vi "Dispatch PVMonitors.vi"(8 "Error In":errorcluster, 11 "CS++ControllerActor in":refnum<class "CS++ControllerActor.lvclass">) -> (0 "Error Out":errorcluster, 3 "CS++ControllerActor out":refnum<class "CS++ControllerActor.lvclass">)   [LabVIEW 2014, in "CS++ControllerActor.lvlib" / "CS++ControllerActor.lvclass"]
doc: "Dispatch nested PVMonitor actors according to PV protocoll prefix."
uses:
  CS++ControllerActor.lvclass
  CS++PVMonitor/CS++PVMonitor.lvclass
  CS++GUIActor Messages/Update-PV Msg/Update-PV Msg.lvclass
  CS++BaseActor/CS++BaseActor.lvclass/CS++BaseActor.ctl
  CS++PVMonitor Messages/CS++PVUpdate Msg/CS++PVUpdate Msg.lvclass/CS++PVUpdate Msg.ctl
  Classes/CS++ProcessVariables/ProcessVariable/PV.lvclass/PV.ctl
  Libraries/Base/FGV Action.ctl
  <vilib>/ActorFramework/Actor/Actor.lvclass/Actor.ctl
  <vilib>/ActorFramework/Message Enqueuer/Message Enqueuer.lvclass/Message Enqueuer.ctl
  CS++ControllerActor.lvclass/CS++ControllerActor.ctl
  CS++PVMonitor Messages/Register PVs Msg/Register PVs Msg.lvclass/Register PVs Msg.ctl
  <vilib>/ActorFramework/Message Enqueuer/Init from Existing Queue.vi
  <vilib>/ActorFramework/Message Enqueuer/Enqueue.vi
  <vilib>/ActorFramework/Message Priority Queue/Priority Enqueue.vi
  CS++PVMonitor Messages/CS++PVUpdate Msg/CS++PVUpdate Msg.lvclass
  Classes/CS++ProcessVariables/PVConnection/PVConnection.lvclass
  Classes/CS++ProcessVariables/ProcessVariable/PV.lvclass
  <vilib>/ActorFramework/Message Enqueuer/Message Enqueuer.lvclass
  CS++PVMonitor Messages/Register PVs Msg/Register PVs Msg.lvclass
  CS++BaseActor/CS++BaseActor.lvclass
  <vilib>/ActorFramework/Actor/Actor.lvclass
  Libraries/Base/CS++Base.lvlib
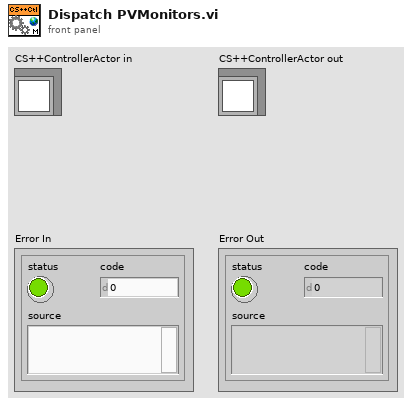
[diagram p1: front panel]
types:
  T1 = cluster{"Msgs":refnum<class "Update-PV Msg.lvclass">[]}[]
  T2 = typedef "CS++Base.lvlib/FGV Action.ctl" = enum16{"add", "replace", "read", "remove", "reset", "get attributes"}
  T3 = cluster{"Name":string, "Polling-String":string, "CS++PVUpdate Msg":refnum<class "CS++PVUpdate Msg.lvclass">, "PVConnection":refnum<class "PVConnection.lvclass">}[]
  T4 = cluster{"Msgs":refnum<class "CS++PVUpdate Msg.lvclass">[]}
  T5 = cluster{"Msgs":refnum<class "CS++PVUpdate Msg.lvclass">[]}[]
  T6 = cluster{refnum<class "CS++PVUpdate Msg.lvclass">[]}
  T7 = cluster{"Accessors:Device Actor's Enqueuer":refnum<class "Message Enqueuer.lvclass">, "Msgs":refnum<class "CS++PVUpdate Msg.lvclass">[]}
  T8 = cluster{"Self Enqueuer":refnum<class "Message Enqueuer.lvclass">, "Msgs":refnum<class "CS++PVUpdate Msg.lvclass">[]}
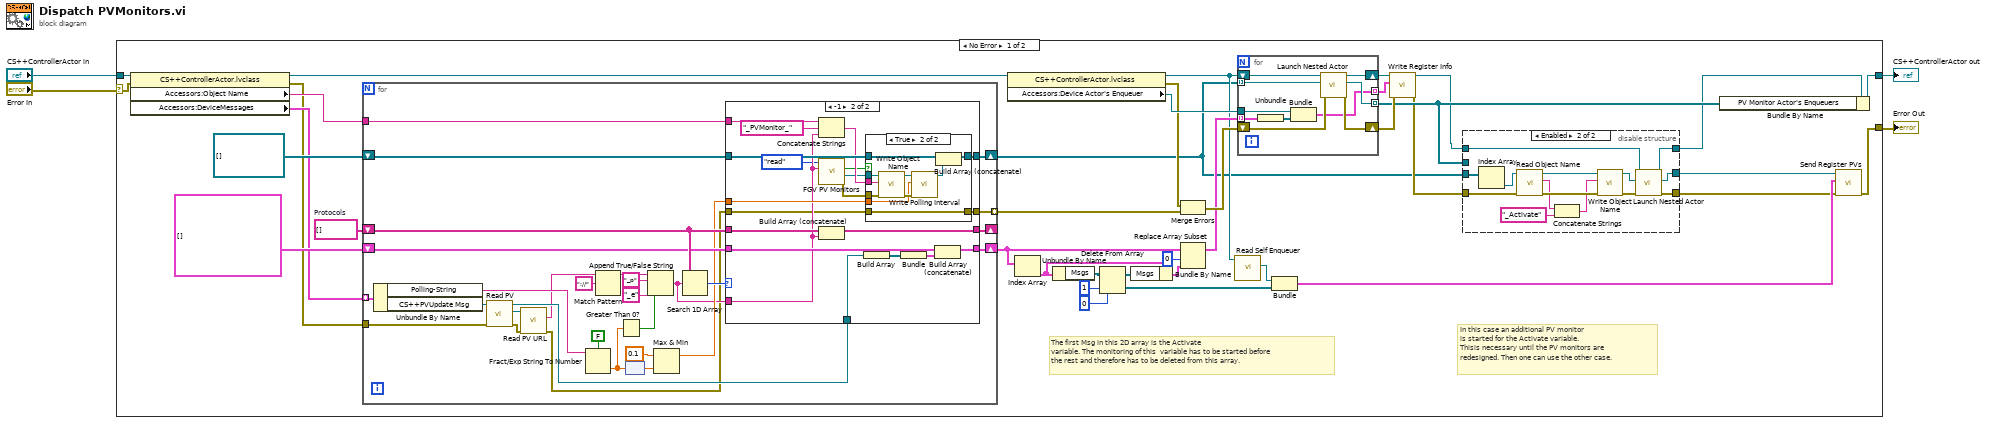
[diagram p0: block diagram]
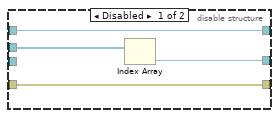
[diagram p2: hidden frame]
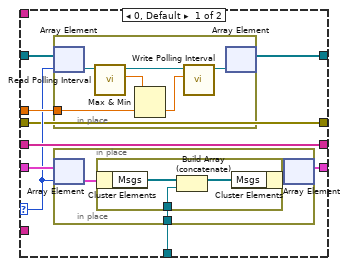
[diagram p3: hidden frame]
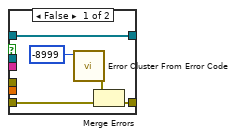
[diagram p4: hidden frame]
diagram:
  n1 = case shown="No Error" "Error In" {
    selector: "Error In" -> [w40 w157]
    tunnel: [w26 w157] -> w3
    tunnel: [w41 w156] -> w1
    tunnel: "CS++ControllerActor in" -> [w42 w156]
    frame No Error {
      w38 = string[] []  # Protocols
      # "In this case an additional PV monitor\nis started for the Activate variable.\nThisis necessary until the PV monitors are\nredesigned. Then one can use the other case."
      # "The first Msg in this 2D array is the Activate\nvariable. The monitoring of this  variable has to be started before\nthe rest and therefore has to be deleted from this array."
      n2 = property class="CS++ControllerActor.lvclass"(reference=w42, error in=w40) -> (reference out=w31:refnum<class "CS++ControllerActor.lvclass">, error out=w29:errorcluster, "Accessors:Object Name"=w34:string, "Accessors:DeviceMessages"=w30:T3)
      n3 = for {
        shift-right: [w99] -> w5
        shift-left: refnum<class "CS++PVMonitor.lvclass">[] [] -> [w96]
        shift-right: [w98] -> _
        shift-left: w38 -> [w97]
        tunnel: w34 -> [w95]
        shift-right: [w93] -> w18
        shift-left: T1 [] -> [w94]
        tunnel: [w92] -> w35 mode=indexing
        tunnel: w30 -> [w79] mode=indexing
        tunnel: w29 -> [w71]
        n4 = Unbundle By Name(w79) -> ("Polling-String"=w78:string, "CS++PVUpdate Msg"=w77:refnum<class "CS++PVUpdate Msg.lvclass">)
        n5 = call "Read PV.vi"("error in (no error)"=w71, "CS++PVUpdate Msg in"=w77) -> ("error out"=w73:errorcluster, "PV"=w75:refnum<class "PV.lvclass">, "CS++PVUpdate Msg out"=w76:refnum<class "CS++PVUpdate Msg.lvclass">)  [unwired: 7 in]
        n6 = call "Read PV URL.vi"("error in (no error)"=w73, "PV in"=w75) -> ("error out"=w72:errorcluster, "PV URL"=w74:string)  [unwired: 7 in, 1 out]
        n7 = Fract/Exp String To Number(use system decimal point (T)=FALSE, string=w78) -> (number=w86:dbl)  [unwired: 2 in, 1 out]
        n8 = Match Pattern(string=w74, regular expression="://") -> (before substring=w84:string)  [unwired: 1 in, 3 out]
        n9 = Greater Than 0?(x=w86) -> (x > 0?=w82:bool)
        n10 = node(w86) -> (w88:dbl[unit])
        n11 = Append True/False String(1:w82, 2:"_e" ("false string"), 3:"_p" ("true string"), 4:w84) -> (0:w83:string)
        n12 = Max & Min(x=dbl[unit] 0.1, y=w88) -> (max(x,y)=w85:dbl[unit])  [unwired: 1 out]
        n13 = Search 1D Array(1D array=w97, element=w83) -> (index of element=w89:i32)  [unwired: 1 in]
        n14 = case shown="-1" w89 {
          selector: w89 -> [w103 _]
          tunnel: [w106 w140] -> w99
          tunnel: [w108 w139] -> w98
          tunnel: w83 -> [_ w127]
          tunnel: w97 -> [w108 w138]
          tunnel: w96 -> [w107 w137]
          tunnel: w85 -> [w105 w134]
          tunnel: w95 -> [_ w133]
          tunnel: w76 -> [w102 w132]
          tunnel: w94 -> [w104 w130]
          tunnel: [w101 w128] -> w93
          tunnel: w72 -> [w100 w123]
          tunnel: [w100 w121] -> w92
          frame 0, Default {
            n15 = in-place {
              in-place-border: w105 -> [w118]
              n16 = in-place-array #1(w107, w103) -> (w120:refnum<class "CS++PVMonitor.lvclass">)
              n17 = call "Read Polling Interval.vi"("CS++BaseActor in"=w120) -> ("Polling Interval"=w119:dbl[unit], "CS++BaseActor out"=w117:refnum<class "CS++PVMonitor.lvclass">)  [unwired: 8 in, 1 out]
              n18 = Max & Min(x=w119, y=w118) -> (min(x,y)=w116:dbl[unit])  [unwired: 1 out]
              n19 = call "Write Polling Interval.vi"("Polling Interval"=w116, "CS++BaseActor in"=w117) -> ("CS++BaseActor out"=w115:refnum<class "CS++PVMonitor.lvclass">)  [unwired: 8 in, 1 out]
              n20 = in-place-array #1(w115) -> (w106:refnum<class "CS++PVMonitor.lvclass">[])  [unwired: 1 out]
            }
            n21 = in-place {
              in-place-border: w102 -> [w109]
              n22 = in-place-array #2(w104, w103) -> (w111:T4)
              n23 = in-place {
                in-place-border: w109 -> [w113]
                n24 = in-place-cluster #3(w111) -> ("Msgs"=w114:refnum<class "CS++PVUpdate Msg.lvclass">[])
                n25 = Build Array (concatenate)(w114, w113) -> (w112:refnum<class "CS++PVUpdate Msg.lvclass">[])
                n26 = in-place-cluster #3("Msgs"=w112) -> (w110:T4)
              }
              n27 = in-place-array #2(w110) -> (w101:T5)  [unwired: 1 out]
            }
          }
          frame -1 {
            n28 = Concatenate Strings(w133, "_PVMonitor_" ("Object Name"), w127) -> (w135:string)
            n29 = call "FGV PV Monitors.vi"("PV Monitor"=w127, "Action (read)"=FGV_Action."read") -> ("Error Out"=w124:errorcluster, "CS++PVMonitor"=w126:refnum<class "CS++PVMonitor.lvclass">, "Success"=w122:bool)  [unwired: 5 in, 2 out]
            n30 = Build Array (concatenate)(w138, w127) -> (w139:string[])
            n31 = Build Array(w132) -> (w131:refnum<class "CS++PVUpdate Msg.lvclass">[])
            n32 = case shown="True" w122 {
              tunnel: [w145 w155] -> w140
              tunnel: w137 -> [w145 w154]
              tunnel: w135 -> [_ w153]
              tunnel: w134 -> [_ w150]
              tunnel: w126 -> [_ w148]
              tunnel: w124 -> [_ w147]
              tunnel: w123 -> [w144 w146]
              tunnel: [w143 w146] -> w121
              frame False {
                n33 = call <vilib>:"Error Cluster From Error Code.vi"("error code (0)"=-8999) -> ("error out"=w142:errorcluster)  [unwired: 8 in]
                n34 = Merge Errors(w142, w144) -> (w143:errorcluster)
              }
              frame True {
                n35 = call "Write Object Name.vi"("error in (no error)"=w147, "Object Name"=w153, "CS++BaseActor in"=w148) -> ("error out"=w151:errorcluster, "CS++BaseActor out"=w152:refnum<class "CS++PVMonitor.lvclass">)  [unwired: 7 in]
                n36 = call "Write Polling Interval.vi"("error in (no error)"=w151, "Polling Interval"=w150, "CS++BaseActor in"=w152) -> ("CS++BaseActor out"=w149:refnum<class "CS++PVMonitor.lvclass">)  [unwired: 7 in, 1 out]
                n37 = Build Array (concatenate)(w154, w149) -> (w155:refnum<class "CS++PVMonitor.lvclass">[])
              }
            }
            n38 = Bundle(w131) -> (w129:T6)  [unwired: 1 in]
            n39 = Build Array (concatenate)(w130, w129) -> (w128:T5)
          }
        }
      }
      n40 = property class="CS++ControllerActor.lvclass"(reference=w31) -> (reference out=w14:refnum<class "CS++ControllerActor.lvclass">, error out=w32:errorcluster, "Accessors:Device Actor's Enqueuer"=w33:refnum<class "Message Enqueuer.lvclass">)  [unwired: 1 in]
      n41 = Index Array(array=w18) -> (element=w20:T4)  [unwired: 1 in]
      n42 = Unbundle By Name(w20) -> ("Msgs"=w22:refnum<class "CS++PVUpdate Msg.lvclass">[])
      n43 = Delete From Array(array=w22, length=1, index=0) -> (deleted portion=w12:refnum<class "CS++PVUpdate Msg.lvclass">[], array with subset deleted=w19:refnum<class "CS++PVUpdate Msg.lvclass">[])
      n44 = Bundle By Name(cluster=w20, "Msgs"=w19) -> (w17:T4)
      n45 = Merge Errors(w32, w35) -> (w37:errorcluster)
      n46 = Replace Array Subset(array=w18, new element=w17, index=0) -> (w15:T5)
      n47 = call <vilib>:"Read Self Enqueuer.vi"("Actor"=w14) -> ("Self Enqueuer"=w13:refnum<class "Message Enqueuer.lvclass">)  [unwired: 10 in]
      n48 = for {
        tunnel: w33 -> [w70]
        tunnel: w5 -> [w66] mode=indexing
        tunnel: w15 -> [w68] mode=indexing
        tunnel: [w64] -> w25 mode=indexing
        shift-right: [w62] -> w27
        shift-left: w37 -> [w69]
        shift-right: [w63] -> w28
        shift-left: w14 -> [w67]
        tunnel: [w61] -> w23 mode=indexing
        n49 = Unbundle(w68) -> ("Msgs"=w65:refnum<class "CS++PVUpdate Msg.lvclass">[])
        n50 = Bundle("Accessors:Device Actor's Enqueuer"=w70, "Msgs"=w65) -> (w61:T7)  [unwired: 1 in]
        n51 = call <vilib>:"Launch Nested Actor.vi"("error in (no error)"=w69, "Nested Actor"=w66, "Caller Actor in"=w67) -> ("error out"=w62:errorcluster, "Nested Actor's Enqueuer"=w64:refnum<class "Message Enqueuer.lvclass">, "Caller Actor out"=w63:refnum<class "CS++ControllerActor.lvclass">)  [unwired: 6 in]
      }
      n52 = Bundle("Self Enqueuer"=w13, "Msgs"=w12) -> (w10:T8)  [unwired: 1 in]
      n53 = call "Write Register Info.vi"("error in (no error)"=w27, "Register Info"=w23, "CS++ControllerActor in"=w28) -> ("error out"=w9:errorcluster, "CS++ControllerActor out"=w7:refnum<class "CS++ControllerActor.lvclass">)  [unwired: 7 in]
      n54 = disable-structure shown="Enabled" {
        disable-tunnel: w25 -> [w46 _]
        disable-tunnel: [w45 w60] -> w24
        disable-tunnel: w9 -> [w44 w50]
        disable-tunnel: [w44 w59] -> w8
        disable-tunnel: w7 -> [w43 w58]
        disable-tunnel: [w43 w57] -> w6
        disable-tunnel: w5 -> [_ w54]
        frame Disabled {
          n55 = Index Array(array=w46) -> (element=w45:refnum<class "Message Enqueuer.lvclass">)  [unwired: 1 in]
        }
        frame Enabled {
          n56 = Index Array(array=w54) -> (element=w51:refnum<class "CS++PVMonitor.lvclass">)  [unwired: 1 in]
          n57 = call "Read Object Name.vi"("error in (no error)"=w50, "CS++BaseActor in"=w51) -> ("error out"=w53:errorcluster, "Object Name"=w48:string, "CS++BaseActor out"=w52:refnum<class "CS++PVMonitor.lvclass">)  [unwired: 7 in]
          n58 = Concatenate Strings(w48, "_Activate" ("string")) -> (w49:string)
          n59 = call "Write Object Name.vi"("error in (no error)"=w53, "Object Name"=w49, "CS++BaseActor in"=w52) -> ("error out"=w56:errorcluster, "CS++BaseActor out"=w55:refnum<class "CS++PVMonitor.lvclass">)  [unwired: 7 in]
          n60 = call <vilib>:"Launch Nested Actor.vi"("error in (no error)"=w56, "Nested Actor"=w55, "Caller Actor in"=w58) -> ("error out"=w59:errorcluster, "Nested Actor's Enqueuer"=w60:refnum<class "Message Enqueuer.lvclass">, "Caller Actor out"=w57:refnum<class "CS++ControllerActor.lvclass">)  [unwired: 6 in]
        }
      }
      n61 = Bundle By Name(cluster=w6, "PV Monitor Actor's Enqueuers"=w25) -> (w41:refnum<class "CS++ControllerActor.lvclass">)
      n62 = call "Send Register PVs.vi"("error in (no error)"=w8, "Register Info"=w10, "Message Enqueuer"=w24) -> ("error out"=w26:errorcluster)  [unwired: 7 in, 1 out]
    }
    frame Error {
    }
  }
  "Error Out" <- w3
  "CS++ControllerActor out" <- w1
